vi "Seq Dialog Sunshade Servo Test.vi"(8 "Segment Data":T1) -> (0 "Step Hisitory":string[](array[string]), 2 "Segment Data 2":T1)   [LabVIEW 2018]
uses:
  type defs/Sequence Info.ctl
  type defs/17x Sunshade Limts Seq.ctl
panel:
  in  "Check Noise":bool
  in  "End Sample":dbl
  in  "Start Sample":dbl
  in  "Variance Max":dbl
  in  "Avg Max":dbl
  in  "Avg Min":dbl
  in  "Overall Max":dbl
  in  "Overall Min":dbl
  out "String 2":string="Pre Run Station - Glass - Vent Open"
  out "error out":errorcluster
  in  "Description":string
  in  "Save":bool
  in  "Cancel":bool
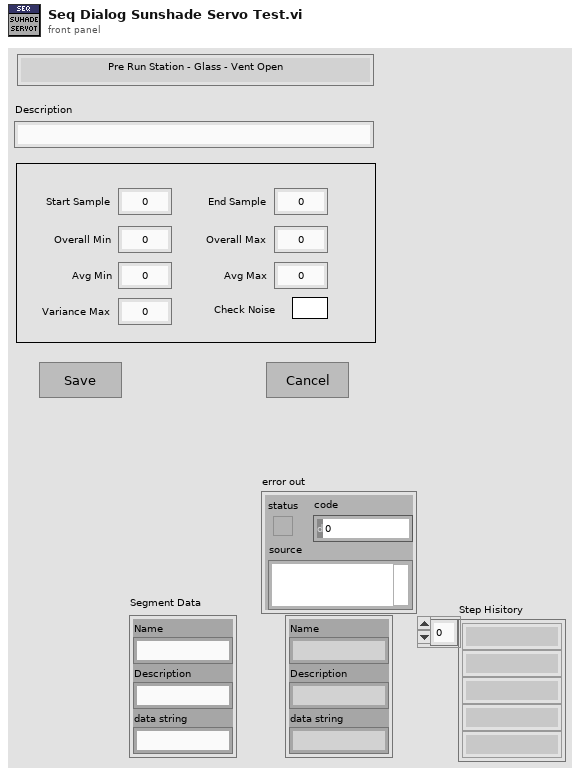
[diagram p1: front panel]
types:
  T1 = typedef "Sequence Info.ctl" = cluster{"Name":string, "Description":string, "data string":string}
  T2 = typedef "17x Sunshade Limts Seq.ctl" = cluster{"Overall Min":dbl, "Overall Max":dbl, "Avg Min":dbl, "Avg Max":dbl, "Truncation Start":dbl, "Truncation End":dbl, "Variance":dbl, "Check Noise":bool}
  T3 = cluster{"Segment Data":T1, "Sun Shade Force Limits":T2, "Old Data":string, "New Data":string}
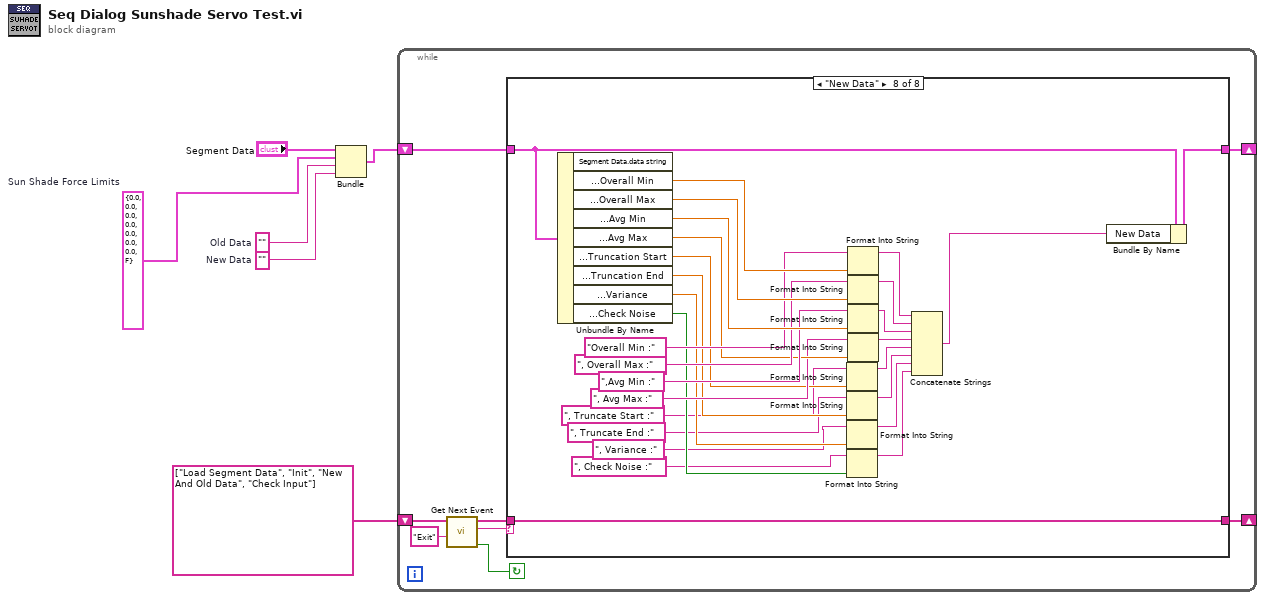
[diagram p0: block diagram]
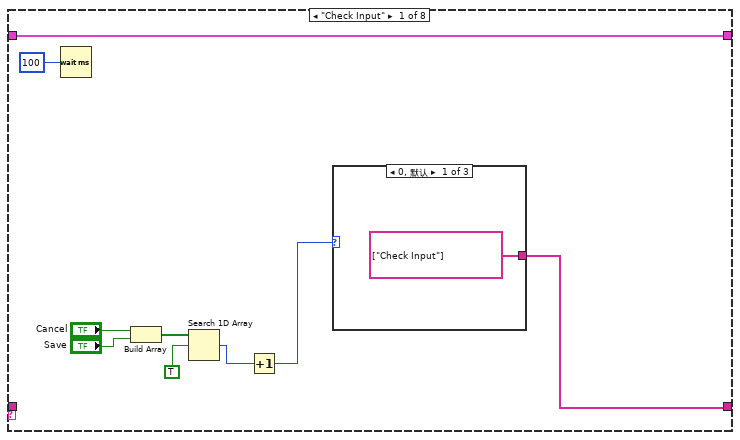
[diagram p2: hidden frame]
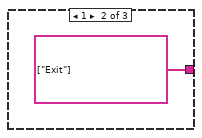
[diagram p3: hidden frame]
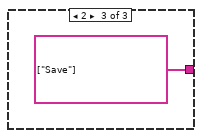
[diagram p4: hidden frame]
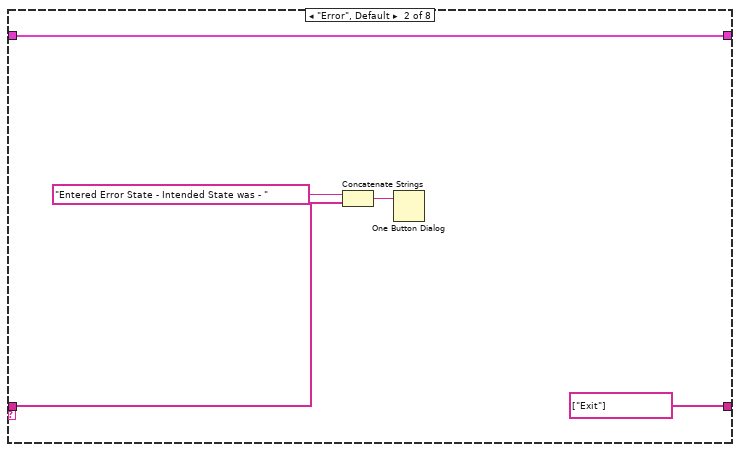
[diagram p5: hidden frame]
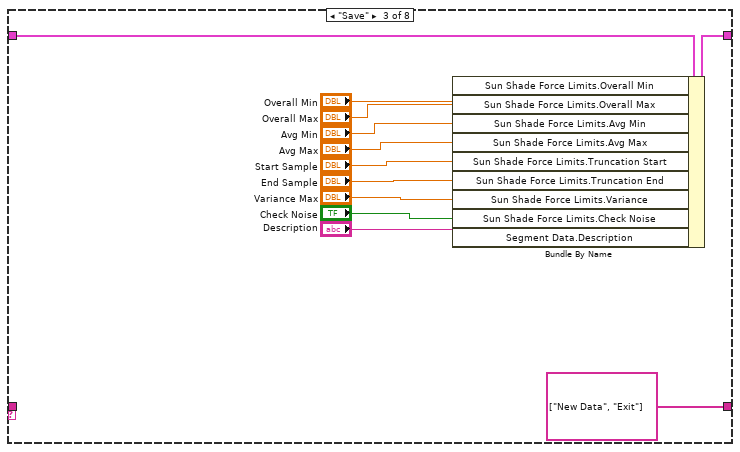
[diagram p6: hidden frame]
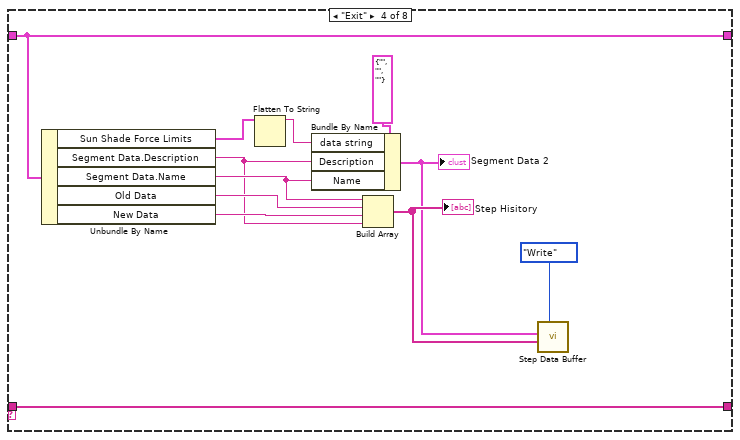
[diagram p7: hidden frame]
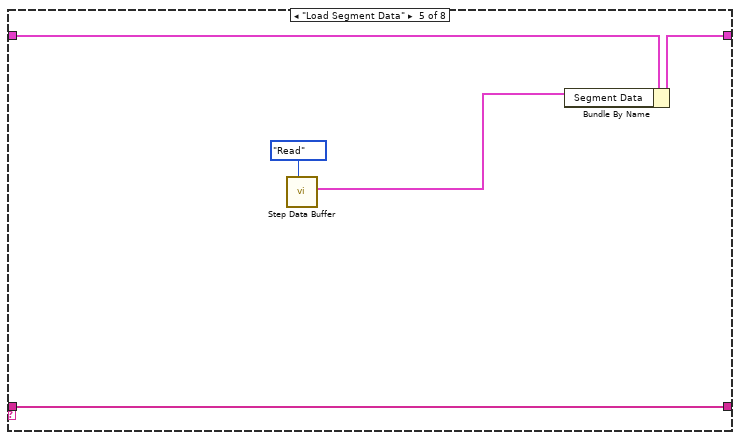
[diagram p8: hidden frame]
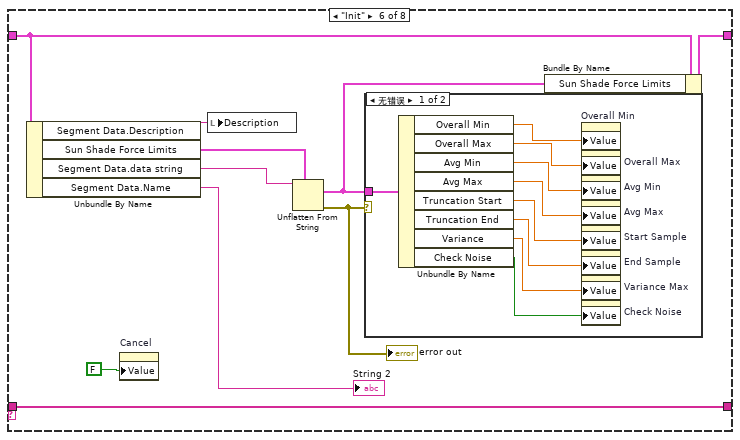
[diagram p9: hidden frame]
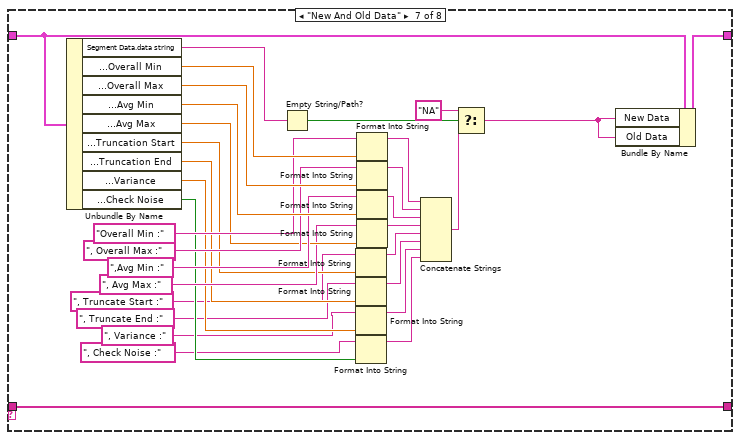
[diagram p11: hidden frame]
diagram:
  w1 = T2 {"Overall Min"=0.0, "Overall Max"=0.0, "Avg Min"=0.0, "Avg Max"=0.0, "Truncation Start"=0.0, "Truncation End"=0.0, "Variance"=0.0, "Check Noise"=FALSE}  # Sun Shade Force Limits
  w3 = ""  # New Data
  w4 = ""  # Old Data
  n1 = Bundle("Segment Data"="Segment Data", "Sun Shade Force Limits"=w1, "Old Data"=w4, "New Data"=w3) -> (w5:T3)  [unwired: 1 in]
  n2 = while {
    shift-right: [w12] -> _
    shift-left: string[] ["Load Segment Data", "Init", "New And Old Data", "Check Input"] ("Event queue out") -> [w11]
    shift-right: [w7] -> _
    shift-left: w5 -> [w8]
    stop <- w10 continue-if-true
    n3 = call "Get Next Event.vi"("Exit Event"="Exit", "event queue in"=w11) -> ("Condition (Exit:F)"=w10:bool, "next event"=w14:string, "event queue out"=w13:string[])  [unwired: 3 in]
    n4 = case shown="\"New Data\"" w14 {
      tunnel: w13 -> [_ w28 _ w55 w60 w70 w111 w115]
      tunnel: [w15 string[] ["Exit"] ("event queue out") string[] ["New Data", "Exit"] ("Event queue out") w55 w60 w70 w111 w115] -> w12
      tunnel: w8 -> [w18 w31 w42 w48 w57 w63 w97 w114]
      tunnel: [w18 w31 w41 w48 w56 w62 w96 w113] -> w7
      frame "Check Input" {
        n5 = Wait (ms)(milliseconds to wait=u32 100) -> ()  [unwired: 1 out]
        n6 = Build Array("Cancel", "Save") -> (w20:bool[])
        n7 = Search 1D Array(1D array=w20, element=TRUE) -> (index of element=w16:i32)  [unwired: 1 in]
        n8 = Increment(x=w16) -> (x+1=w17:i32)
        n9 = case shown="0, 默认" w17 {
          tunnel: [string[] ["Check Input"] ("Events to Insert") string[] ["Exit"] ("Events to Insert") string[] ["Save"] ("Events to Insert")] -> w15
          frame 0, Default {
          }
          frame 1 {
          }
          frame 2 {
          }
        }
      }
      frame "Error", Default {
        n10 = Concatenate Strings("Entered Error State - Intended State was - " ("string"), w28) -> (w29:string)
        n11 = One Button Dialog(message=w29) -> ()  [unwired: 1 in, 1 out]
      }
      frame "Save" {
        n12 = Bundle By Name(cluster=w42, "Sun Shade Force Limits.Overall Min"="Overall Min", "Sun Shade Force Limits.Overall Max"="Overall Max", "Sun Shade Force Limits.Avg Min"="Avg Min", "Sun Shade Force Limits.Avg Max"="Avg Max", "Sun Shade Force Limits.Truncation Start"="Start Sample", "Sun Shade Force Limits.Truncation End"="End Sample", "Sun Shade Force Limits.Variance"="Variance Max", "Sun Shade Force Limits.Check Noise"="Check Noise", "Segment Data.Description"="Description") -> (w41:T3)
      }
      frame "Exit" {
        n13 = Unbundle By Name(w48) -> ("Sun Shade Force Limits"=w54:T2, "Segment Data.Description"=w44:string, "Segment Data.Name"=w49:string, "Old Data"=w51:string, "New Data"=w50:string)
        n14 = Flatten To String(anything=w54) -> (data string=w52:string)  [unwired: 3 in, 2 out]
        n15 = Bundle By Name(cluster=T1 {"Name"="", "Description"="", "data string"=""} ("Segment Data"), "data string"=w52, "Description"=w44, "Name"=w49) -> (w45:T1)
        "Segment Data 2" <- w45
        n16 = Build Array(w49, w51, w50, w44) -> (w46:string[])
        "Step Hisitory" <- w46
        n17 = call "Step Data Buffer.vi"("Mode"=enum16{"Init", "Read", "Write"}."Write", "Step Hisitory In"=w46, "Segment Data In"=w45) -> ()  [unwired: 4 in, 5 out]
      }
      frame "Load Segment Data" {
        n18 = call "Step Data Buffer.vi"("Mode"=enum16{"Init", "Read", "Write"}."Read") -> ("Segment Data Out"=w58:T1)  [unwired: 6 in, 4 out]
        n19 = Bundle By Name(cluster=w57, "Segment Data"=w58) -> (w56:T3)
      }
      frame "Init" {
        n20 = Unbundle By Name(w63) -> ("Segment Data.Description"=w65:string, "Sun Shade Force Limits"=w68:T2, "Segment Data.data string"=w69:string, "Segment Data.Name"=→"String 2":string)
        n21 = property on="Cancel" class="Bool (严格)"("Value"=FALSE ("Cancel")) -> ()  [unwired: 2 in, 2 out]
        n22 = local write "Description"(w65) -> ()
        n23 = Unflatten From String(type=w68, binary string=w69) -> (value=w64:T2, error out=w67:errorcluster)  [unwired: 3 in, 1 out]
        "error out" <- w67
        n24 = case shown="无错误" w67 {
          tunnel: w64 -> [w79 _]
          frame No Error {
            n25 = Unbundle By Name(w79) -> ("Overall Min"=w78:dbl, "Overall Max"=w77:dbl, "Avg Min"=w76:dbl, "Avg Max"=w75:dbl, "Truncation Start"=w74:dbl, "Truncation End"=w73:dbl, "Variance"=w72:dbl, "Check Noise"=w71:bool)
            n26 = property on="Overall Min" class="DigNum (严格)"("Value"=w78) -> ()  [unwired: 2 in, 2 out]
            n27 = property on="Overall Max" class="DigNum (严格)"("Value"=w77) -> ()  [unwired: 2 in, 2 out]
            n28 = property on="Avg Min" class="DigNum (严格)"("Value"=w76) -> ()  [unwired: 2 in, 2 out]
            n29 = property on="Avg Max" class="DigNum (严格)"("Value"=w75) -> ()  [unwired: 2 in, 2 out]
            n30 = property on="Start Sample" class="DigNum (严格)"("Value"=w74) -> ()  [unwired: 2 in, 2 out]
            n31 = property on="End Sample" class="DigNum (严格)"("Value"=w73) -> ()  [unwired: 2 in, 2 out]
            n32 = property on="Variance Max" class="DigNum (严格)"("Value"=w72) -> ()  [unwired: 2 in, 2 out]
            n33 = property on="Check Noise" class="Bool (严格)"("Value"=w71) -> ()  [unwired: 2 in, 2 out]
          }
          frame Error {
          }
        }
        n34 = Bundle By Name(cluster=w63, "Sun Shade Force Limits"=w64) -> (w62:T3)
      }
      frame "New And Old Data" {
        n35 = Unbundle By Name(w97) -> ("Segment Data.data string"=w110:string, "Sun Shade Force Limits.Overall Min"=w105:dbl, "Sun Shade Force Limits.Overall Max"=w103:dbl, "Sun Shade Force Limits.Avg Min"=w101:dbl, "Sun Shade Force Limits.Avg Max"=w93:dbl, "Sun Shade Force Limits.Truncation Start"=w91:dbl, "Sun Shade Force Limits.Truncation End"=w90:dbl, "Sun Shade Force Limits.Variance"=w89:dbl, "Sun Shade Force Limits.Check Noise"=w88:bool)
        n36 = Empty String/Path?(string/path=w110) -> (empty?=w109:bool)
        n37 = Format Into String(initial string=", Truncate Start :" ("string"), w91) -> (resulting string=w87:string)  [unwired: 2 in, 1 out]
        n38 = Format Into String(initial string=", Truncate End :" ("string"), w90) -> (resulting string=w86:string)  [unwired: 2 in, 1 out]
        n39 = Format Into String(initial string=", Variance :" ("string"), w89) -> (resulting string=w85:string)  [unwired: 2 in, 1 out]
        n40 = Format Into String(initial string=", Check Noise :" ("string"), w88) -> (resulting string=w84:string)  [unwired: 2 in, 1 out]
        n41 = Format Into String(initial string="Overall Min :" ("string"), w105) -> (resulting string=w104:string)  [unwired: 2 in, 1 out]
        n42 = Format Into String(initial string=", Overall Max :" ("string"), w103) -> (resulting string=w102:string)  [unwired: 2 in, 1 out]
        n43 = Format Into String(initial string=",Avg Min :" ("string"), w101) -> (resulting string=w95:string)  [unwired: 2 in, 1 out]
        n44 = Format Into String(initial string=", Avg Max :" ("string"), w93) -> (resulting string=w94:string)  [unwired: 2 in, 1 out]
        n45 = Concatenate Strings(w104, w102, w95, w94, w87, w86, w85, w84) -> (w106:string)
        n46 = Select(t="NA", s=w109, f=w106) -> (s? t:f=w107:string)
        n47 = Bundle By Name(cluster=w97, "New Data"=w107, "Old Data"=w107) -> (w96:T3)
      }
      frame "New Data" {
        n48 = Unbundle By Name(w114) -> ("Sun Shade Force Limits.Overall Min"=w139:dbl, "Sun Shade Force Limits.Overall Max"=w137:dbl, "Sun Shade Force Limits.Avg Min"=w135:dbl, "Sun Shade Force Limits.Avg Max"=w129:dbl, "Sun Shade Force Limits.Truncation Start"=w127:dbl, "Sun Shade Force Limits.Truncation End"=w126:dbl, "Sun Shade Force Limits.Variance"=w125:dbl, "Sun Shade Force Limits.Check Noise"=w124:bool)  [unwired: 1 out]
        n49 = Format Into String(initial string=", Truncate Start :" ("string"), w127) -> (resulting string=w123:string)  [unwired: 2 in, 1 out]
        n50 = Format Into String(initial string=", Truncate End :" ("string"), w126) -> (resulting string=w122:string)  [unwired: 2 in, 1 out]
        n51 = Format Into String(initial string=", Variance :" ("string"), w125) -> (resulting string=w121:string)  [unwired: 2 in, 1 out]
        n52 = Format Into String(initial string=", Check Noise :" ("string"), w124) -> (resulting string=w120:string)  [unwired: 2 in, 1 out]
        n53 = Format Into String(initial string="Overall Min :" ("string"), w139) -> (resulting string=w138:string)  [unwired: 2 in, 1 out]
        n54 = Format Into String(initial string=", Overall Max :" ("string"), w137) -> (resulting string=w136:string)  [unwired: 2 in, 1 out]
        n55 = Format Into String(initial string=",Avg Min :" ("string"), w135) -> (resulting string=w131:string)  [unwired: 2 in, 1 out]
        n56 = Format Into String(initial string=", Avg Max :" ("string"), w129) -> (resulting string=w130:string)  [unwired: 2 in, 1 out]
        n57 = Concatenate Strings(w138, w136, w131, w130, w123, w122, w121, w120) -> (w112:string)
        n58 = Bundle By Name(cluster=w114, "New Data"=w112) -> (w113:T3)
      }
    }
  }
